vi "Analog PWM In.vi"() -> ()   [LabVIEW 2019]
uses:
  Submodules/Source/Types/PWM.Measure.Analog.Measurement.ctl
  <vilib>/rvi/Emulation/niFpgaGetClockAttributes.vi
  <vilib>/rvi/Emulation/niFpgaSctlEmulationGetInTimedLoop.vi
  <vilib>/rvi/Emulation/niFpgaEmulationReportErrorSimple.vi
  <vilib>/rvi/Emulation/niFpgaCriticalErrorInLSC.vi
  Submodules/Source/Speciality FPGA IO.lvlib
panel:
  in  "INACTIVE VOLTAGE":fxp<+/-,32,8>
  in  "ACTIVE VOLTAGE":fxp<+/-,32,8>
  in  "ACQ TICKS":u32
  in  "INACTIVE TICKS":u32
  in  "ACTIVE TICKS":u32
  out "Analog PWM In":T1
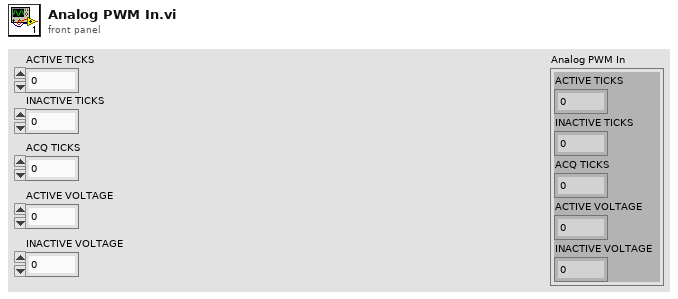
[diagram p1: front panel]
types:
  T1 = typedef "Speciality FPGA IO.lvlib/PWM.Measure.Analog.Measurement.ctl" = cluster{"ACTIVE TICKS":u32, "INACTIVE TICKS":u32, "ACQ TICKS":u32, "ACTIVE VOLTAGE":fxp<+/-,32,8>, "INACTIVE VOLTAGE":fxp<+/-,32,8>}
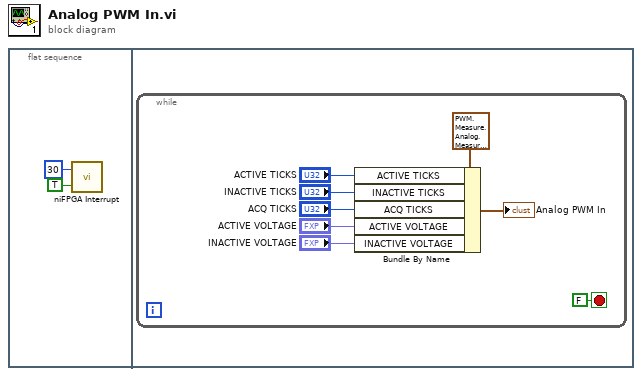
[diagram p0: block diagram]
diagram:
  n1 = flat-sequence {
    frame #0 {
      n2 = call <vilib>:"niFPGA Interrupt.vi"("Wait Until Cleared (F)"=TRUE, "IRQ Number (0)"=u8 30) -> ()  [unwired: 1 in]
    }
    frame #1 {
      n3 = while {
        stop <- FALSE stop-if-true
        n4 = Bundle By Name(cluster=T1 {"ACTIVE TICKS"=0, "INACTIVE TICKS"=0, "ACQ TICKS"=0, "ACTIVE VOLTAGE"=0.0, "INACTIVE VOLTAGE"=0.0}, "ACTIVE TICKS"="ACTIVE TICKS", "INACTIVE TICKS"="INACTIVE TICKS", "ACQ TICKS"="ACQ TICKS", "ACTIVE VOLTAGE"="ACTIVE VOLTAGE", "INACTIVE VOLTAGE"="INACTIVE VOLTAGE") -> (→"Analog PWM In":T1)
      }
    }
  }
